vi "Integral action.vi"(0 "derivative action":dbl format="%.2f", 3 "proportional action":dbl format="%.2f", 5 "prev. control output":dbl format="%.2f", 6 "options":T1={"sp low"=0.0, "sp high"=100.0, "out low"=-100.0, "out high"=100.0, "hold (F)"=FALSE, "auto (T)"=TRUE, "pro. band (F)"=FALSE, "reverse acting (T)"=TRUE, "beta"=1.0, "linearity"=1.0, "dt (s)"=-1.0} {"dt (s)" format="%.2f"; "linearity" min=0.0 max=1.0 format="%.2f"; "sp low" format="%.2f"; "sp high" format="%.2f"; "out low" format="%.2f"; "out high" format="%.2f"; "beta" min=0.0 max=1.0 format="%.2f"}, 7 "PID parameters":cluster{"Kp":dbl, "Ti":dbl, "Td":dbl} {"Td" format="%.2f"; "Ti" format="%.2f"; "Kp" format="%.2f"}, 8 "iteration":i32, 9 "dt":dbl format="%.2f", 10 "error":dbl format="%.2f", 11 "Ki":dbl format="%.4f") -> (2 "integral action":dbl format="%.2f")   [LabVIEW 2020, in "NI_PID__prctrl compat.lvlib"]
doc: "This function calculates the integral action of the PID controller.\n\nA non-linear term is added to the integral action to avoid integrator windup when error values are very large. The term used is:\n\n1 / (1 + (10 * e^2 / sp_range^2))\n\nTherefore a large error will cause the integral action to be reduced to approximately 10%. When the error is 0, the integral action is 100%.\n\nThis VI also compensates for any change in control parameters (such as PID gains) by correcting the integrated error term to ensure smooth controller output. This method is used to prevent integrator windup when the controller output is saturated."
uses:
  <vilib>/addons/control/pid/NI_PID__prctrl compat.lvlib
panel:
  # "Proportional gain or band (Kc)"
  # "Integral (reset) time (Ti, min)"
  # "Derivative (rate) time (Td, min)"
  # "SP & PV range:"
  # "Output range:"
  # "-1: default,using\nsystem clock"
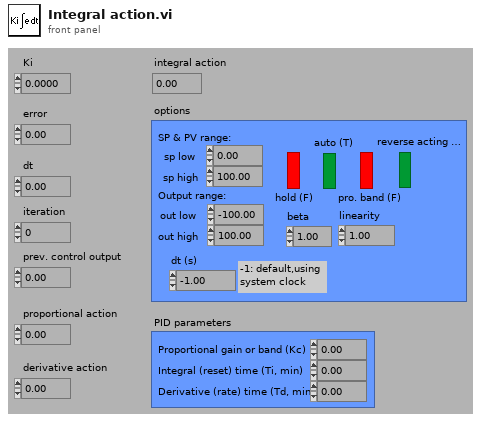
[diagram p1: front panel]
types:
  T1 = cluster{"sp low":dbl, "sp high":dbl, "out low":dbl, "out high":dbl, "hold (F)":bool, "auto (T)":bool, "pro. band (F)":bool, "reverse acting (T)":bool, "beta":dbl, "linearity":dbl, "dt (s)":dbl}
  T2 = cluster{"sp low":bool, "sp high":bool, "out low":bool, "out high":bool, "hold (F)":bool, "auto (T)":bool, "pro. band (F)":bool, "reverse acting (T)":bool, "beta":bool, "linearity":bool, "dt (s)":bool}
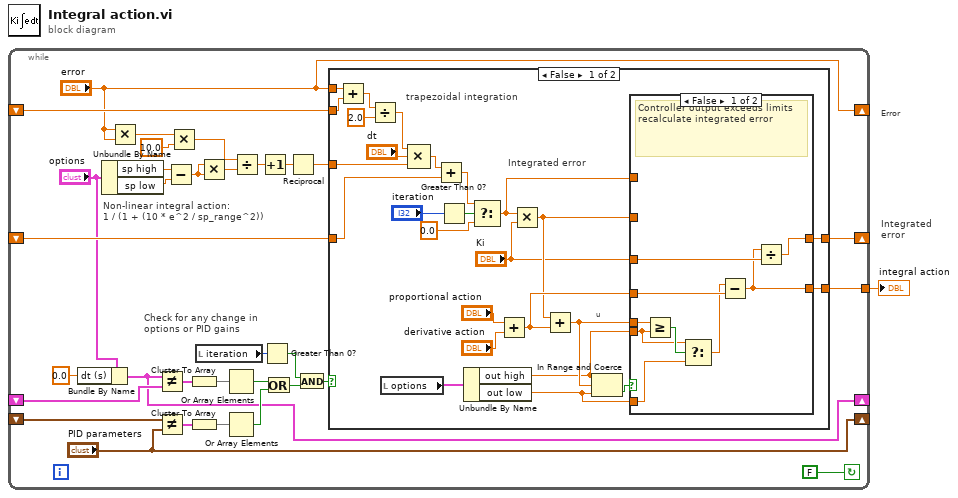
[diagram p0: block diagram]
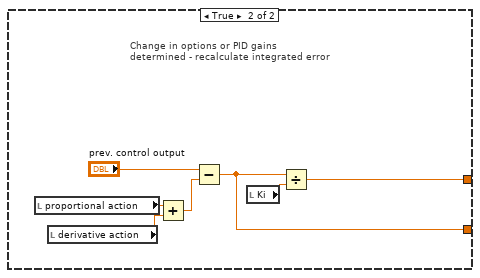
[diagram p3: hidden frame]
diagram:
  # "Integrated\nerror"
  # "Error"
  n1 = while {
    tunnel: [w4] -> w1
    shift-left: _ -> [w3]
    shift-right: ["PID parameters"] -> _
    shift-left: _ -> [w22]
    shift-right: [w21] -> _
    shift-left: _ -> [w32]
    shift-right: [w31] -> _
    shift-left: _ -> [w33]
    shift-right: ["error"] -> _
    stop <- FALSE continue-if-true
    # "Non-linear integral action:\n1 / (1 + (10 * e^2 / sp_range^2))"
    # "Check for any change in\noptions or PID gains"
    n2 = Bundle By Name(cluster="options", "dt (s)"=0.0) -> (w21:T1)
    n3 = Unbundle By Name("options") -> ("sp high"=w20:dbl, "sp low"=w19:dbl)
    n4 = Multiply(x="error", y="error") -> (x*y=w14:dbl)
    n5 = Not Equal?(x=w21, y=w22) -> (x != y?=w25:T2)
    n6 = Not Equal?(x=w3, y="PID parameters") -> (x != y?=w28:cluster{"Kp":bool, "Ti":bool, "Td":bool})
    n7 = Subtract(x=w20, y=w19) -> (x-y=w12:dbl)
    n8 = Multiply(x=w14, y=10.0) -> (x*y=w17:dbl)
    n9 = Cluster To Array(cluster=w25) -> (array=w26:bool[])
    n10 = Cluster To Array(cluster=w28) -> (array=w27:bool[])
    n11 = local read "iteration"() -> (w6:i32)
    n12 = Multiply(x=w12, y=w12) -> (x*y=w13:dbl)
    n13 = Or Array Elements(Boolean array=w26) -> (logical OR=w29:bool)
    n14 = Or Array Elements(Boolean array=w27) -> (logical OR=w30:bool)
    n15 = Divide(x=w17, y=w13) -> (x/y=w16:dbl)
    n16 = Increment(x=w16) -> (x+1=w15:dbl)
    n17 = Greater Than 0?(x=w6) -> (x > 0?=w5:bool)
    n18 = Or(x=w29, y=w30) -> (x .or. y?=w8:bool)
    n19 = Reciprocal(x=w15) -> (1/x=w10:dbl)
    n20 = And(x=w5, y=w8) -> (x .and. y?=w7:bool)
    n21 = case shown="False" w7 {
      tunnel: "error" -> [w59 _]
      tunnel: [w46 w74] -> w31
      tunnel: w32 -> [w57 _]
      tunnel: w33 -> [w49 _]
      tunnel: w10 -> [w34 _]
      tunnel: [w36 w73] -> w4
      frame False {
        # "u"
        # "trapezoidal integration"
        # "Integrated error"
        n22 = Add(x=w59, y=w49) -> (x+y=w50:dbl)
        n23 = Divide(x=w50, y=2.0) -> (x/y=w52:dbl)
        n24 = local read "options"() -> (w47:T1)
        n25 = Compound Arithmetic op=MULTIPLY(w52, "dt", w34) -> (w56:dbl)
        n26 = Add(x=w56, y=w57) -> (x+y=w58:dbl)
        n27 = Greater Than 0?(x="iteration") -> (x > 0?=w54:bool)
        n28 = Unbundle By Name(w47) -> ("out high"=w43:dbl, "out low"=w42:dbl)
        n29 = Select(t=w58, s=w54, f=0.0) -> (s? t:f=w41:dbl)
        n30 = Add(x="proportional action", y="derivative action") -> (x+y=w38:dbl)
        n31 = Multiply(x=w41, y="Ki") -> (x*y=w37:dbl)
        n32 = Add(x=w37, y=w38) -> (x+y=w44:dbl)
        n33 = In Range and Coerce(upper limit=w43, x=w44, lower limit=w42) -> (In Range?=w45:bool)  [unwired: 1 out]
        n34 = case shown="False" w45 {
          tunnel: w41 -> [_ w69]
          tunnel: [w62 w69] -> w46
          tunnel: w44 -> [w68 _]
          tunnel: w43 -> [w66 _]
          tunnel: w42 -> [w65 _]
          tunnel: "Ki" -> [w63 _]
          tunnel: w38 -> [w64 _]
          tunnel: [w61 w70] -> w36
          tunnel: w37 -> [_ w70]
          frame False {
            # "Controller output exceeds limits\nrecalculate integrated error"
            n35 = Greater Or Equal?(x=w68, y=w66) -> (x >= y?=w67:bool)
            n36 = Select(t=w66, s=w67, f=w65) -> (s? t:f=w60:dbl)
            n37 = Subtract(x=w60, y=w64) -> (x-y=w61:dbl)
            n38 = Divide(x=w61, y=w63) -> (x/y=w62:dbl)
          }
          frame True {
            # "Controller output within\nspecified range"
          }
        }
      }
      frame True {
        # "Change in options or PID gains\ndetermined - recalculate integrated error"
        n39 = local read "proportional action"() -> (w77:dbl)
        n40 = local read "derivative action"() -> (w76:dbl)
        n41 = Add(x=w77, y=w76) -> (x+y=w75:dbl)
        n42 = Subtract(x="prev. control output", y=w75) -> (x-y=w73:dbl)
        n43 = local read "Ki"() -> (w72:dbl)
        n44 = Divide(x=w73, y=w72) -> (x/y=w74:dbl)
      }
    }
  }
  "integral action" <- w1
